vi "Get BlockNode ImageData.vi"(8 "error in (no error)":errorcluster, 11 "steering type (\"\")":string) -> (0 "error out":errorcluster, 3 "image data":T1)   [LabVIEW 2017, in "NI_Robotics_Create Steering Frame.xnode"]
uses:
  <vilib>/robotics/Steering/Create Steering Frame/NI_Robotics_Create Steering Frame.xnode
  <vilib>/picture/picture.llb/imagedata.ctl
  <vilib>/XNodeSupport/XNodeImage.ctl
  <vilib>/XNodeSupport/NI_XNodeSupport.lvlib
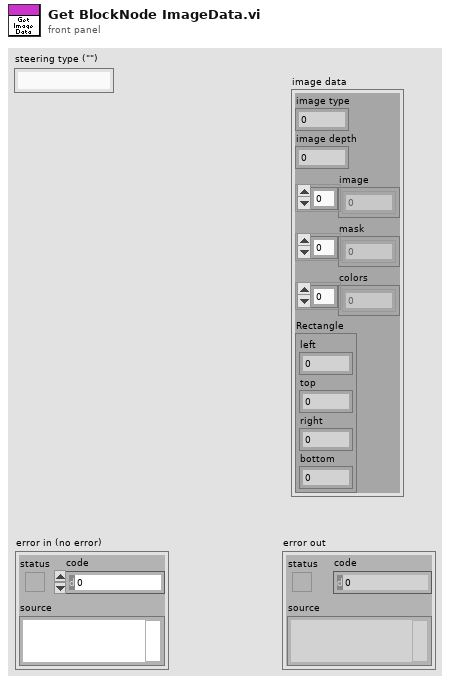
[diagram p1: front panel]
types:
  T1 = typedef "imagedata.ctl" = cluster{"image type":i32, "image depth":i32, "image":u8[], "mask":u8[], "colors":u32[], "Rectangle":cluster{"left":i16, "top":i16, "right":i16, "bottom":i16}}
  T2 = typedef "NI_XNodeSupport.lvlib/XNodeImage.ctl" = picture
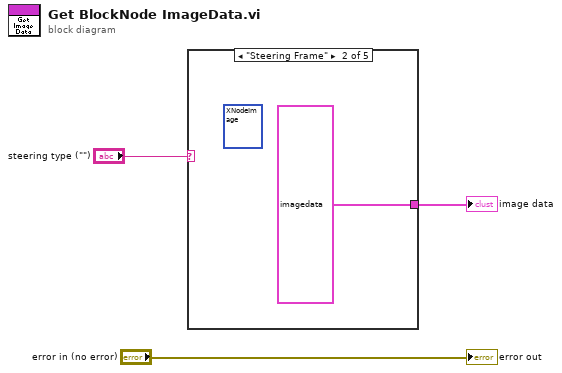
[diagram p0: block diagram]
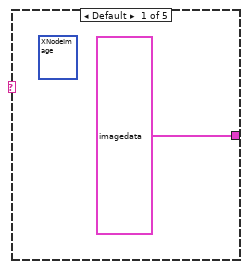
[diagram p2: hidden frame]
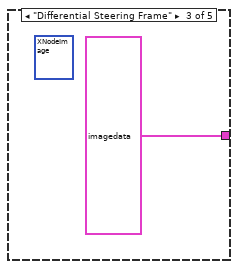
[diagram p3: hidden frame]
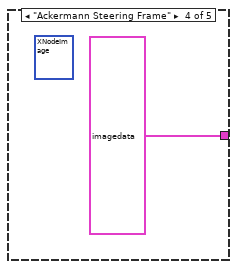
[diagram p4: hidden frame]
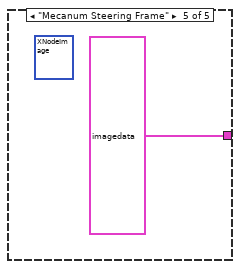
[diagram p5: hidden frame]
diagram:
  n1 = case shown="\"Steering Frame\"" "steering type (\"\")" {
    tunnel: [T1 {"image type"=0, "image depth"=24, "image"=array[3072 elements], "mask"=[], "colors"=[], "Rectangle"={"left"=0, "top"=0, "right"=32, "bottom"=32}} ("image data") T1 {"image type"=0, "image depth"=24, "image"=array[3072 elements], "mask"=[], "colors"=[], "Rectangle"={"left"=0, "top"=0, "right"=32, "bottom"=32}} ("image data") T1 {"image type"=0, "image depth"=24, "image"=array[3072 elements], "mask"=[], "colors"=[], "Rectangle"={"left"=0, "top"=0, "right"=32, "bottom"=32}} ("image data") T1 {"image type"=0, "image depth"=24, "image"=array[3072 elements], "mask"=[], "colors"=[], "Rectangle"={"left"=0, "top"=0, "right"=32, "bottom"=32}} ("image data") T1 {"image type"=0, "image depth"=24, "image"=array[3072 elements], "mask"=[], "colors"=[], "Rectangle"={"left"=0, "top"=0, "right"=32, "bottom"=32}} ("image data")] -> w1
    frame Default {
      (unwired) T2 bytes[3102] ("Image")
    }
    frame "Steering Frame" {
      (unwired) T2 bytes[3102] ("Image")
    }
    frame "Differential Steering Frame" {
      (unwired) T2 bytes[3102] ("Image")
    }
    frame "Ackermann Steering Frame" {
      (unwired) T2 bytes[3102] ("Image")
    }
    frame "Mecanum Steering Frame" {
      (unwired) T2 bytes[3102] ("Image")
    }
  }
  "image data" <- w1
  "error out" <- "error in (no error)"
